vi "2-Main Reference calculation.vi"() -> ()   [LabVIEW 2015]
uses:
  <vilib>/Utility/file.llb/Read Delimited Spreadsheet (string).vi
  <vilib>/Utility/file.llb/Write Delimited Spreadsheet (string).vi
panel:
  out "output":dbl[](array[numeric])
  out "Current process of inter cycles":i32
  out "Number of inter cycles":i32
  out "Current process of external cycles":i32
  out "Number of external cycles":i32
  out "imageWidth":i32=700
  in  "waveLengthSample":i32=1004
  in  "waveLengthNumber":i32=250
  out "Files under current path":string[](array[string])
  out "Current binary":string
  out "Current path":string
  in  "Save path":path=path "I:/2017 Maize-Hyper-Program/2017 Maize Test sample/Result"
  in  "Binary path":path=path "I:/2017 Maize-Hyper-Program/2017 Maize Test sample/path.txt"
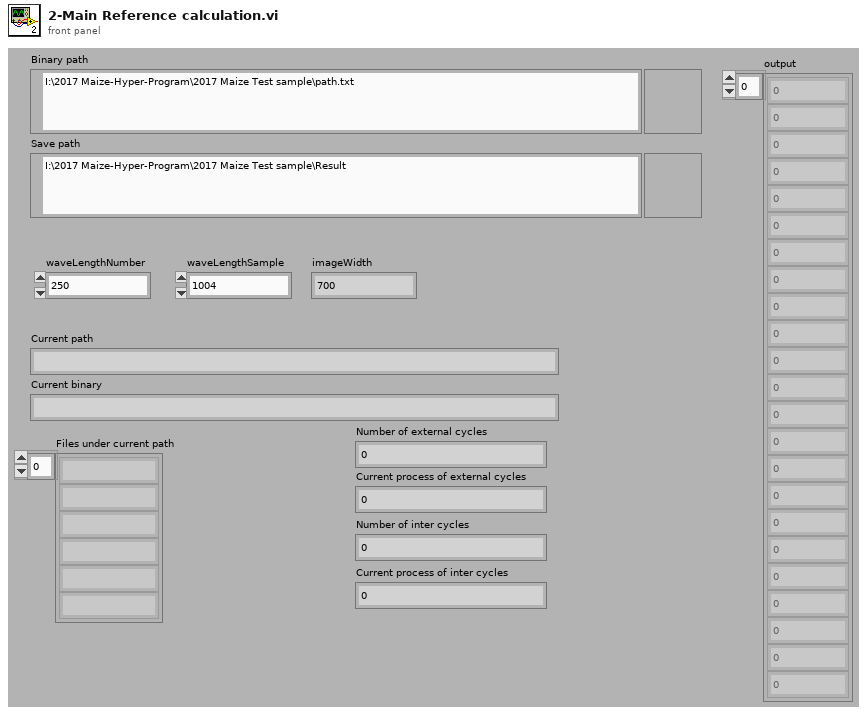
[diagram p1: front panel]
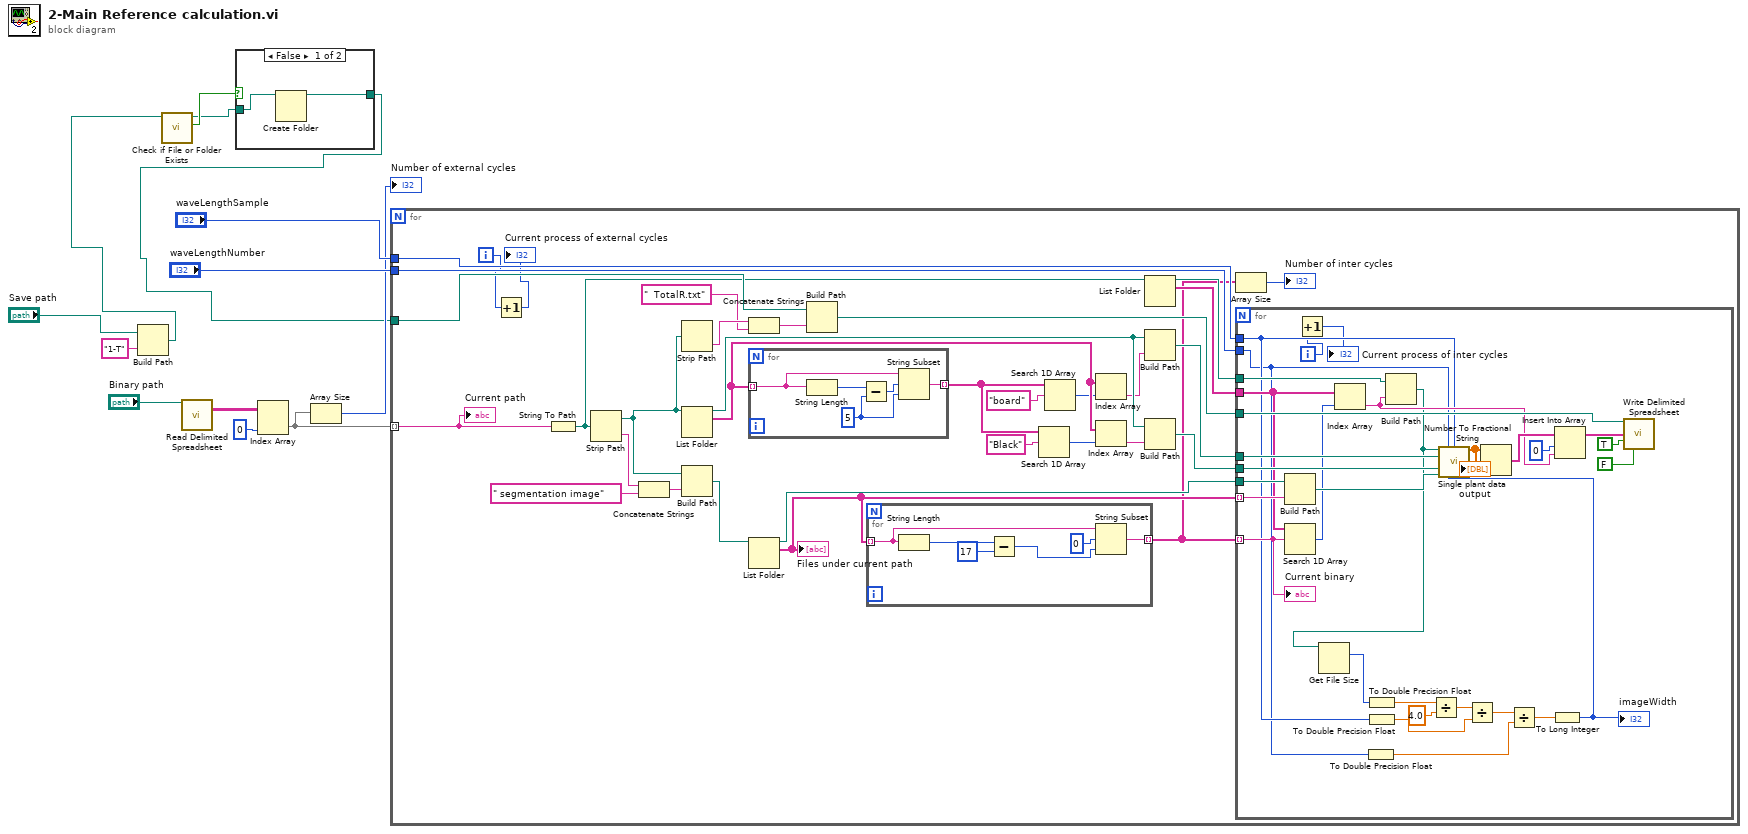
[diagram p0: block diagram]
diagram:
  n1 = Build Path(base path="Save path", name or relative path="1-T") -> (appended path=w4:path)
  n2 = call <vilib>:"Check if File or Folder Exists.vi"("path"=w4) -> ("file or folder exists?"=w3:bool, "dup path"=w2:path)  [unwired: 8 in, 1 out]
  n3 = call-poly <vilib>:"Read Delimited Spreadsheet.vi"("file path (dialog if empty)"="Binary path") -> ("all rows"=w11:string[][])  [unwired: 9 in, 5 out]
  n4 = case shown="False" w3 {
    tunnel: w2 -> [w15 w16]
    tunnel: [w14 w16] -> w1
    frame False {
      n5 = Create Folder(path (use dialog)=w15) -> (created path=w14:path)  [unwired: 2 in, 2 out]
    }
    frame True {
    }
  }
  n6 = Index Array(array=w11, index (col)=0 ("disabled index (col)")) -> (element=w8:string[])  [unwired: 1 in]
  n7 = Array Size(array=w8) -> (size(s)=→"Number of external cycles":i32)
  n8 = for {
    tunnel: w8 -> [w49] mode=indexing
    tunnel: w1 -> [w43]
    tunnel: "waveLengthNumber" -> [w24]
    tunnel: "waveLengthSample" -> [w23]
    i -> [w18]
    n9 = Increment(x=w18) -> (x+1=→"Current process of external cycles":i32)
    n10 = String To Path(string=w49) -> (path=w40:path)
    n11 = Strip Path(path=w40) -> (stripped path=w19:path, name=w47:string)
    n12 = Concatenate Strings(w47, " segmentation image" ("string")) -> (w46:string)
    n13 = Strip Path(path=w19) -> (name=w45:string)  [unwired: 1 out]
    n14 = List Folder(path=w19) -> (path out=w28:path, filenames=w32:string[])  [unwired: 3 in, 2 out]
    n15 = Build Path(base path=w19, name or relative path=w46) -> (appended path=w41:path)
    n16 = Concatenate Strings(w45, "  TotalR.txt" ("string")) -> (w42:string)
    n17 = for {
      tunnel: w32 -> [w54] mode=indexing
      tunnel: [w50] -> w35 mode=indexing
      w52 = 5 ("length (rest)")
      n18 = String Length(string=w54) -> (length=w53:i32)
      n19 = Subtract(x=w53, y=w52) -> (x-y=w51:i32)
      n20 = String Subset(string=w54, offset (0)=w51, length (rest)=w52) -> (substring=w50:string)
    }
    n21 = List Folder(path=w41) -> (path out=w37:path, filenames=w38:string[])  [unwired: 1 in, 4 out]
    "Files under current path" <- w38
    n22 = Build Path(base path=w43, name or relative path=w42) -> (appended path=w36:path)
    n23 = for {
      tunnel: w38 -> [w91] mode=indexing
      tunnel: [w87] -> w20 mode=indexing
      n24 = String Length(string=w91) -> (length=w89:i32)
      n25 = Subtract(x=w89, y=17) -> (x-y=w88:i32)
      n26 = String Subset(string=w91, offset (0)=0, length (rest)=w88) -> (substring=w87:string)
    }
    n27 = Search 1D Array(1D array=w35, element="Black") -> (index of element=w31:i32)  [unwired: 1 in]
    n28 = Search 1D Array(1D array=w35, element="board") -> (index of element=w30:i32)  [unwired: 1 in]
    n29 = Index Array(array=w32, index=w30) -> (element=w27:string)
    n30 = Index Array(array=w32, index=w31) -> (element=w29:string)
    n31 = List Folder(path=w40) -> (path out=w39:path, filenames=w22:string[])  [unwired: 1 in, 4 out]
    n32 = Build Path(base path=w28, name or relative path=w27) -> (appended path=w26:path)
    n33 = Build Path(base path=w28, name or relative path=w29) -> (appended path=w25:path)
    n34 = Array Size(array=w20) -> (size(s)=→"Number of inter cycles":i32)
    n35 = for {
      tunnel: w39 -> [w85]
      tunnel: w22 -> [w72]
      tunnel: w20 -> [w74] mode=indexing
      tunnel: w38 -> [w73] mode=indexing
      tunnel: w37 -> [w84]
      tunnel: w36 -> [w81]
      tunnel: w26 -> [w78]
      tunnel: w25 -> [w77]
      tunnel: w24 -> [w61]
      tunnel: w23 -> [w62]
      i -> [w57]
      n36 = Build Path(base path=w84, name or relative path=w73) -> (appended path=w76:path)
      n37 = Search 1D Array(1D array=w72, element=w74) -> (index of element=w71:i32)  [unwired: 1 out]
      n38 = Increment(x=w57) -> (x+1=→"Current process of inter cycles":i32)
      n39 = Index Array(array=w72, index=w71) -> (element=w70:string)
      n40 = To Double Precision Float(number=w61) -> (double precision float=w59:dbl)
      n41 = To Double Precision Float(number=w62) -> (double precision float=w60:dbl)
      n42 = Build Path(base path=w85, name or relative path=w70) -> (appended path=w64:path)
      n43 = Get File Size(file=w64) -> (size (in bytes)=w63:i64)  [unwired: 1 in, 2 out]
      n44 = To Double Precision Float(number=w63) -> (double precision float=w65:dbl)
      n45 = Divide(x=w65, y=4.0) -> (x/y=w67:dbl)
      n46 = Divide(x=w67, y=w60) -> (x/y=w68:dbl)
      n47 = Divide(x=w68, y=w59) -> (x/y=w69:dbl)
      n48 = To Long Integer(number=w69) -> (32bit integer=w58:i32)
      "imageWidth" <- w58
      n49 = call "Single plant data.vi"("binarypath"=w64, "waveLengthNumber"=w61, "waveLengthSample"=w62, "whitepath"=w78, "blackpath"=w77, "imagepath"=w76, "imageWidth"=w58) -> ("output"=w55:dbl[])  [unwired: 8 in]
      "output" <- w55
      n50 = Number To Fractional String(number=w55) -> (F-format string=w83:string[])  [unwired: 3 out]
      n51 = Insert Into Array(array=w83, index=0, new element=w70) -> (w79:string[])
      n52 = call-poly <vilib>:"Write Delimited Spreadsheet.vi"("file path (dialog if empty)"=w81, "1D data"=w79, "append to file? (F)"=TRUE, "transpose? (F)"=FALSE ("append to file? (new file:F)")) -> ()  [unwired: 10 in, 2 out]
      "Current binary" <- w74
    }
    "Current path" <- w49
  }
